vi "For Loops.vi"() -> ()   [LabVIEW 2019]
panel:
  in  "Numeric 3":i32
  out "number (0 to 1) 2":dbl
  out "Numeric 2":i32
  out "Numeric":i32
  in  "stop":bool
  out "number (0 to 1)":dbl
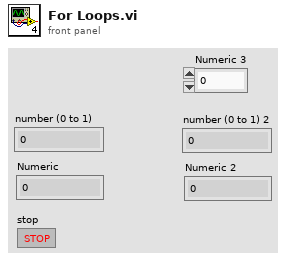
[diagram p1: front panel]
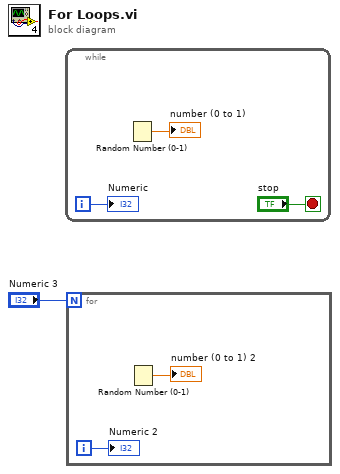
[diagram p0: block diagram]
diagram:
  n1 = while {
    i -> [w2]
    stop <- "stop" stop-if-true
    n2 = Random Number (0-1)() -> (number: 0 to 1=→"number (0 to 1)":dbl)
    "Numeric" <- w2
  }
  n3 = for {
    N: "Numeric 3" -> [_]
    i -> [w5]
    n4 = Random Number (0-1)() -> (number: 0 to 1=→"number (0 to 1) 2":dbl)
    "Numeric 2" <- w5
  }
